vi "Gui_SetupExperimentDefault.vi"(7 "entrée d'erreur (pas d'erreur)":errorcluster, 10 "EXPERIMENT Inputs":T1={"User Name"="", "Date"="", "Comment"="", "Experiment Steps"=[], "Sample Components"=[], "Molecules"=[], "Laser 1"={"Used"=TRUE, "Name"="Spectroscopy", "Reference"="Yag", "Wavelength"=1000.0, "Energy"=25.0}, "Laser 2"={"Used"=TRUE, "Name"="Spectroscopy", "Reference"="Yag", "Wavelength"=1000.0, "Energy"=25.0}, "Laser 3"={"Used"=TRUE, "Name"="Spectroscopy", "Reference"="Yag", "Wavelength"=1000.0, "Energy"=25.0}} caption="EXCIT Paths") -> (0 "sortie d'erreur":errorcluster, 3 "Tableau":string[](array[string]))   [LabVIEW 2015]
uses:
  controls/EXPERIMENT_Inputs.ctl
  controls/LASER_Inputs.ctl
panel:
  out "EXPERIMENT Outputs":T1={"User Name"="", "Date"="", "Comment"="", "Experiment Steps"=[], "Sample Components"=[], "Molecules"=[], "Laser 1"={"Used"=TRUE, "Name"="Spectroscopy", "Reference"="Yag", "Wavelength"=1000.0, "Energy"=25.0}, "Laser 2"={"Used"=TRUE, "Name"="Spectroscopy", "Reference"="Yag", "Wavelength"=1000.0, "Energy"=25.0}, "Laser 3"={"Used"=TRUE, "Name"="Spectroscopy", "Reference"="Yag", "Wavelength"=1000.0, "Energy"=25.0}} caption="EXCIT Paths"
  in  "OK":bool
  in  "Molecules":i32[](listbox)
  # "Name"
  # "Reference"
  # "(nm)"
  # "E (J)"
  # "Laser 1"
  # "Laser 2"
  # "Laser 3"
  # "Name"
  # "Reference"
  # "(nm)"
  # "E (J)"
  # "Laser 1"
  # "Laser 2"
  # "Laser 3"
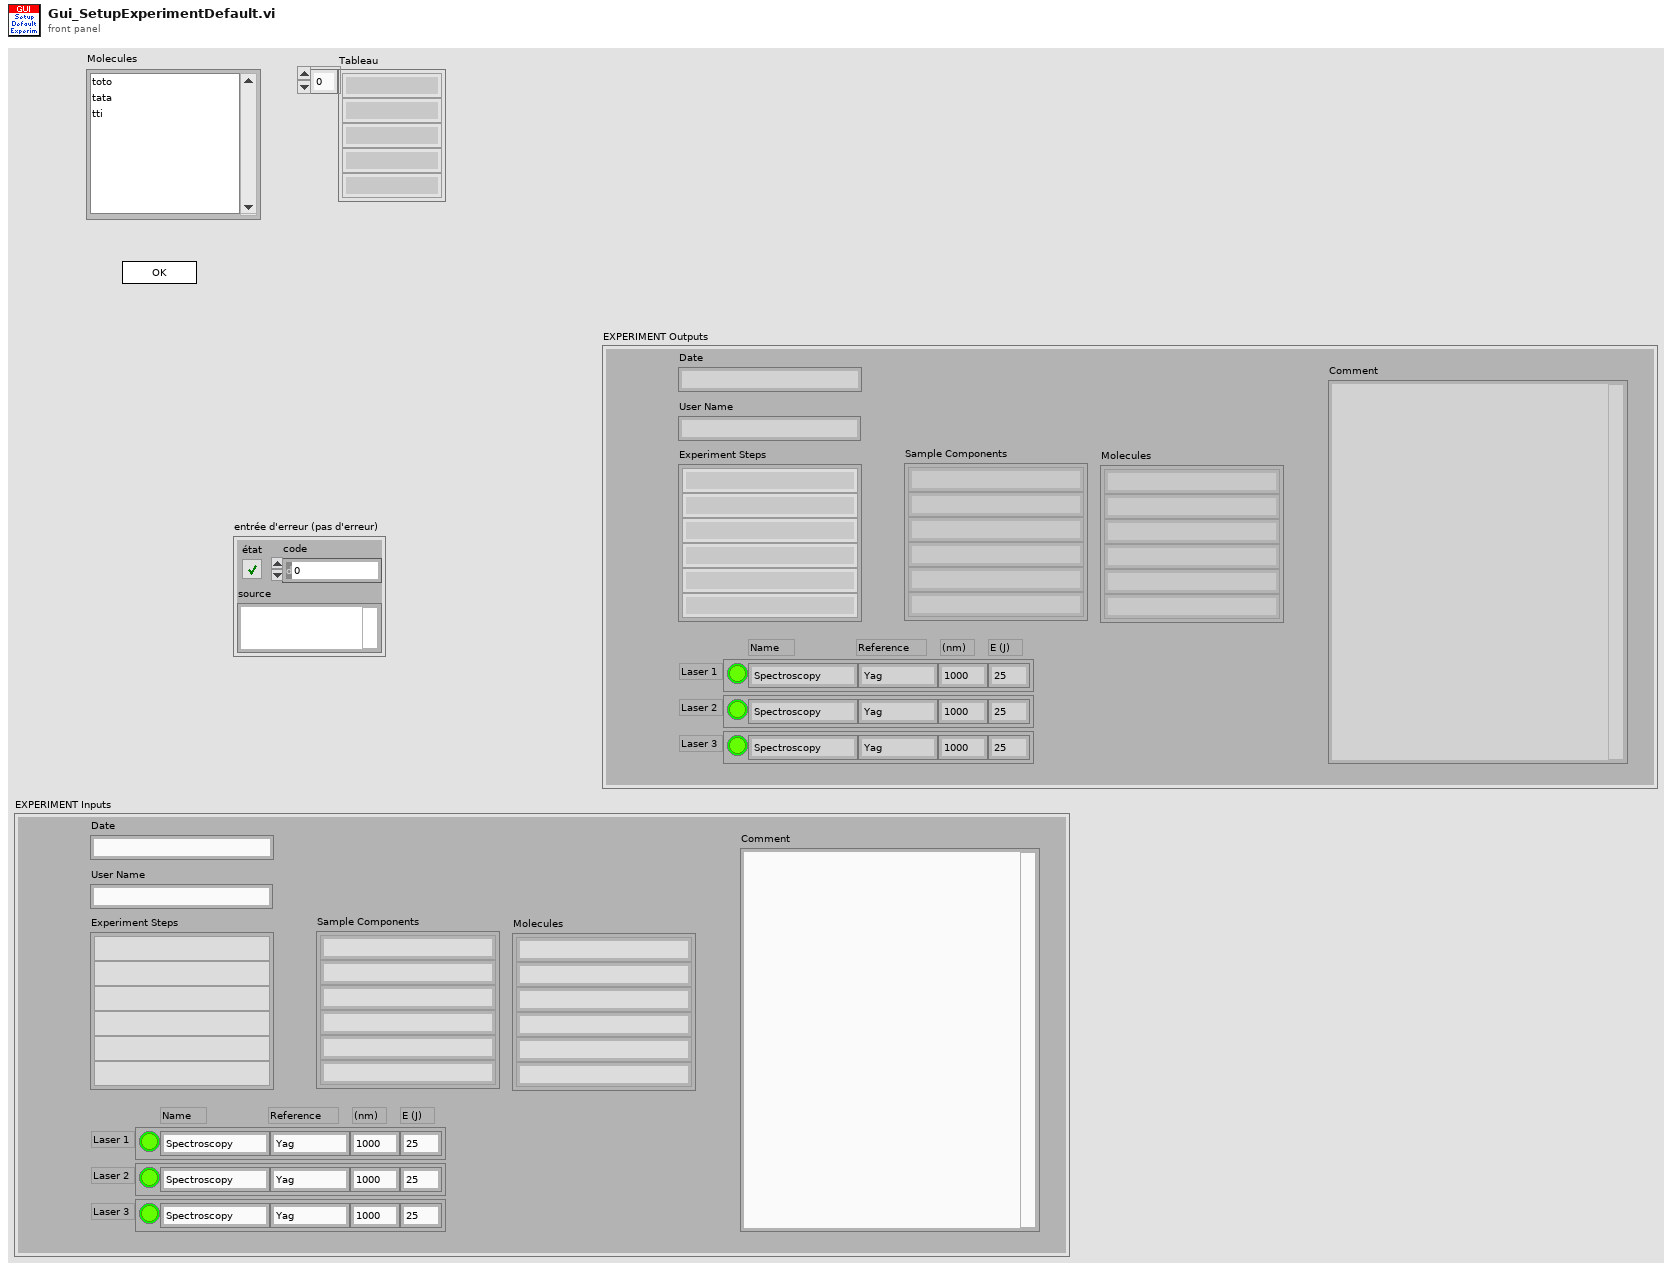
[diagram p1: front panel]
types:
  T1 = typedef "EXPERIMENT_Inputs.ctl" = cluster{"User Name":string, "Date":string, "Comment":string, "Experiment Steps":string[], "Sample Components":string[], "Molecules":string[], "Laser 1":T2, "Laser 2":T2, "Laser 3":T2}
  T2 = typedef "LASER_Inputs.ctl" = cluster{"Used":bool, "Name":string, "Reference":string, "Wavelength":dbl, "Energy":dbl}
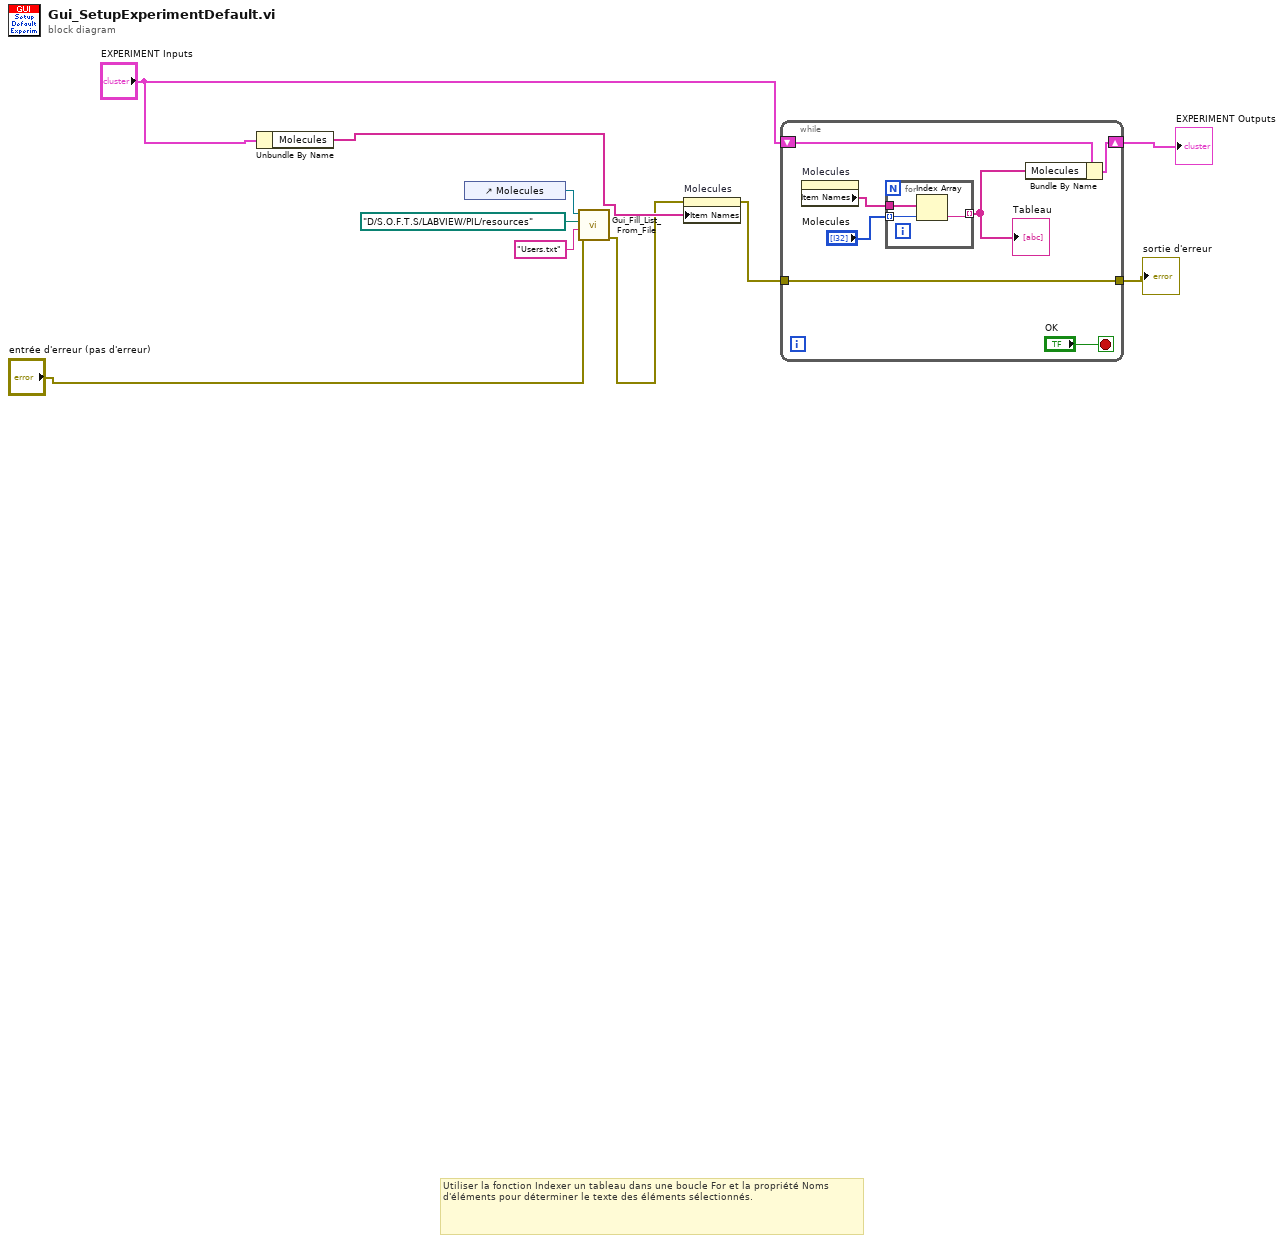
[diagram p0: block diagram]
diagram:
  # "Utiliser la fonction Indexer un tableau dans une boucle For et la propriété Noms d'éléments pour déterminer le texte des éléments sélectionnés."
  n1 = Unbundle By Name("EXPERIMENT Inputs") -> ("Molecules"=w6:string[])
  n2 = control-ref of="Molecules"() -> (w3:refnum<vi>)
  n3 = call "Gui_Fill_List_From_File.vi"("error in (no error)"="entrée d'erreur (pas d'erreur)", "Resource Name"="Users.txt", "Resource Path"=path "D:/S.O.F.T.S/LABVIEW/PIL/resources", "Refnum LstDér"=w3) -> ("error out"=w4:errorcluster)  [unwired: 5 in, 2 out]
  n4 = property on="Molecules" class="LstDér (strict)"(error in=w4, "Item Names"=w6) -> (error out=w10:errorcluster)  [unwired: 1 in, 1 out]
  n5 = while {
    tunnel: w10 -> [w15]
    tunnel: [w15] -> w9
    shift-right: [w12] -> w8
    shift-left: "EXPERIMENT Inputs" -> [w14]
    stop <- "OK" stop-if-true
    n6 = property on="Molecules" class="LstDér (strict)"() -> ("Item Names"=w16:string[])  [unwired: 2 in, 2 out]
    n7 = for {
      tunnel: [w20] -> w13 mode=indexing
      tunnel: w16 -> [w19]
      tunnel: "Molecules" -> [w18] mode=indexing
      n8 = Index Array(array=w19, index=w18) -> (element=w20:string)
    }
    "Tableau" <- w13
    n9 = Bundle By Name(cluster=w14, "Molecules"=w13) -> (w12:T1)
  }
  "sortie d'erreur" <- w9
  "EXPERIMENT Outputs" <- w8
